vi "test_rm_imu.vi"() -> ()   [LabVIEW 2023]
panel:
  out "samples":T1(array[cluster])
  out "pose":sgl[][](array[numeric])
  in  "stop":bool
  in  "host":string="192.168.1.7"
  in  "port":u16=3806
  in  "path in":path=path "C:/Users/jcds/Documents/GitHub/hl2ss/extensions/client_labview/hl2ss_labview/hl2ss_ulm.dll"
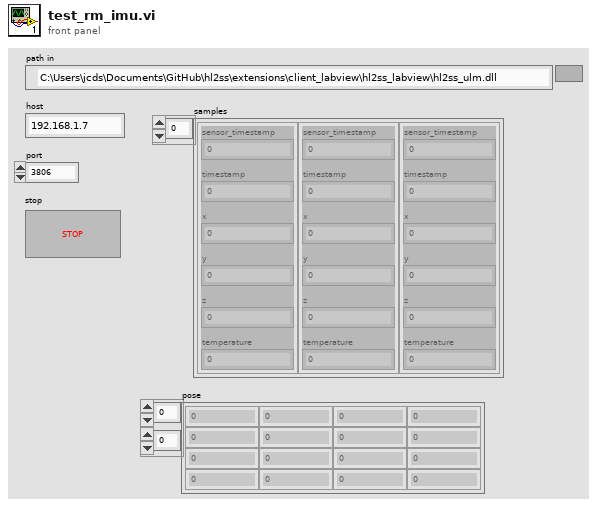
[diagram p1: front panel]
types:
  T1 = cluster{"sensor_timestamp":u64, "timestamp":u64, "x":sgl, "y":sgl, "z":sgl, "temperature":sgl}[]
  T2 = cluster{"chunk":u64, "mode":u8, "_reserved_0":u8, "_reserved_1":u8, "_reserved_2":u8, "_reserved_3":u8, "_reserved_4":u8, "_reserved_5":u8, "_reserved_6":u8}
  T3 = cluster{"frame_stamp":i64, "timestamp":u64, "payload_size":u32, "status":i32, "payload":u64, "pose":u64}
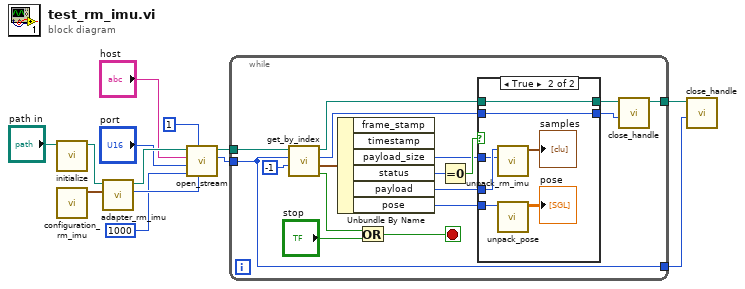
[diagram p0: block diagram]
diagram:
  n1 = call "initialize.vi"("path in"="path in") -> ("path out"=w12:path)  [unwired: 9 in, 1 out]
  n2 = call "configuration_rm_imu.vi"() -> ("configuration_rm_imu"=w13:T2)  [unwired: 11 in]
  n3 = call "adapter_rm_imu.vi"("configuration_rm_imu"=w13, "path in"=w12) -> ("configuration"=w9:u64, "path out"=w10:path)  [unwired: 8 in]
  n4 = call "open_stream.vi"("configuration"=w9, "decoded"=u8 1, "buffer_size"=u64 1000, "port"="port", "host"="host", "path in"=w10) -> ("handle"=w4:u64, "path out"=w5:path)  [unwired: 3 in, 1 out]
  n5 = while {
    tunnel: w5 -> [w30]
    tunnel: w4 -> [w15]
    tunnel: [w16] -> w3
    tunnel: [w15] -> w2
    stop <- w28 stop-if-true
    n6 = call "get_by_index.vi"("frame_stamp"=i64 -1, "stream_handle"=w15, "path in"=w30) -> ("error"=w27:bool, "packet"=w25:T3, "packet_handle"=w19:u64, "path out"=w20:path)  [unwired: 5 in]
    n7 = Unbundle By Name(w25) -> ("payload_size"=w14:u32, "status"=w22:i32, "payload"=w24:u64, "pose"=w23:u64)  [unwired: 2 out]
    n8 = Or(x=w27, y="stop") -> (x .or. y?=w28:bool)
    n9 = Equal To 0?(x=w22) -> (x = 0?=w21:bool)
    n10 = case shown="True" w21 {
      tunnel: w24 -> [_ w35]
      tunnel: w23 -> [_ w39]
      tunnel: w20 -> [w31 w37]
      tunnel: w19 -> [w32 w36]
      tunnel: [w31 w37] -> w18
      tunnel: [w32 w36] -> w17
      tunnel: w14 -> [_ w34]
      frame False {
      }
      frame True {
        n11 = call "unpack_rm_imu.vi"("payload_size"=w34, "payload"=w35) -> ("samples"=→"samples":T1)  [unwired: 8 in, 1 out]
        n12 = call "unpack_pose.vi"("pose"=w39) -> ("pose"=→"pose":sgl[][])  [unwired: 9 in, 1 out]
      }
    }
    n13 = call "close_handle.vi"("handle"=w17, "path in"=w18) -> ("path out"=w16:path)  [unwired: 9 in]
  }
  n14 = call "close_handle.vi"("handle"=w2, "path in"=w3) -> ()  [unwired: 9 in, 1 out]
